vi "Build All VI HTML Documentation.vi"(6 "Requirement":string="Labstache", 7 "Destination":path=path "", 8 "Error In":errorcluster, 11 "Source In":path) -> (0 "Error Out":errorcluster, 3 "Source Out":path)   [LabVIEW 2018, in "Scripts.lvlib"]
uses:
  Scripts.lvlib
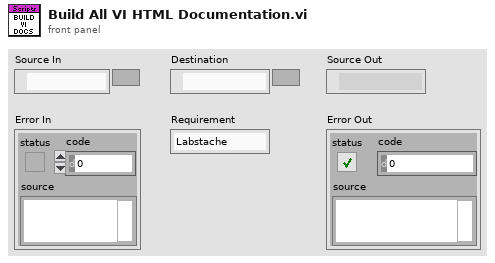
[diagram p1: front panel]
types:
  T1 = enum32{"invalid VI type", "Standard VI", "Control VI", "Global VI", "Polymorphic VI", "Configuration VI", "SubSystem", "Facade VI", "Method VI", "Statechart Diagram VI"}
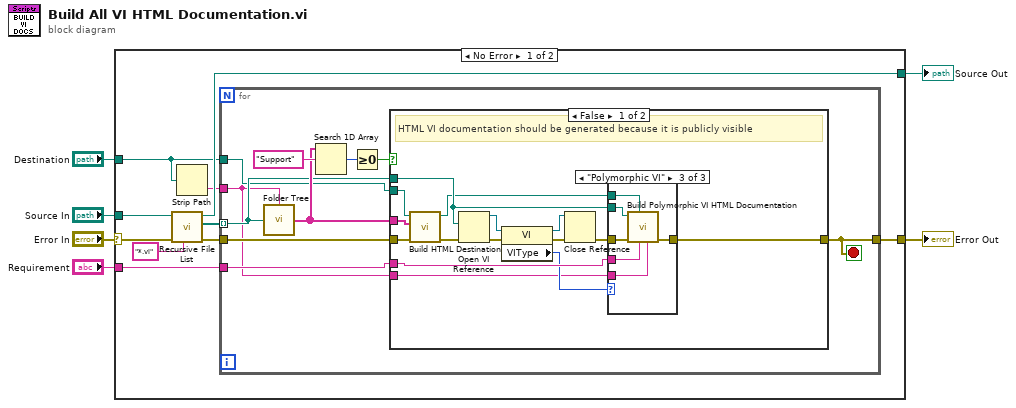
[diagram p0: block diagram]
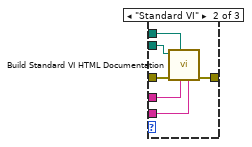
[diagram p3: hidden frame]
diagram:
  n1 = case shown="No Error" "Error In" {
    selector: "Error In" -> [w11 w57]
    tunnel: [w13 w57] -> w6
    tunnel: "Requirement" -> [w12 _]
    tunnel: "Destination" -> [w8 _]
    tunnel: "Source In" -> [w10 w56]
    tunnel: [w9 w56] -> w1
    frame No Error {
      n2 = call <vilib>:"Recursive File List.vi"("pattern"="*.vi", "error in (no error)"=w11, "Folder Path"=w10) -> ("error out"=w14:errorcluster, "All Files in Dir"=w15:path[], "dup Folder Path"=w9:path)  [unwired: 4 in, 2 out]
      n3 = Strip Path(path=w8) -> (name=w7:string)  [unwired: 1 out]
      n4 = for {
        tunnel: w15 -> [w20] mode=indexing
        tunnel: w14 -> [w22]
        tunnel: w7 -> [w18]
        tunnel: [w21] -> w13
        tunnel: w12 -> [w19]
        tunnel: w8 -> [w17]
        stop <- w21 stop-if-true
        n5 = call "Folder Tree.vi"("File"=w20, "Root Folder Name"=w18) -> ("Hierarchy Folders"=w23:string[])
        n6 = Search 1D Array(1D array=w23, element="Support") -> (index of element=w25:i32)  [unwired: 1 in]
        n7 = Greater Or Equal To 0?(x=w25) -> (x >= 0?=w24:bool)
        n8 = case shown="False" w24 {
          tunnel: w23 -> [w40 _]
          tunnel: w22 -> [w41 w55]
          tunnel: [w39 w55] -> w21
          tunnel: w20 -> [w33 _]
          tunnel: w19 -> [w38 _]
          tunnel: w18 -> [w30 _]
          tunnel: w17 -> [w29 _]
          frame False {
            # "HTML VI documentation should be generated because it is publicly visible"
            n9 = call "Build HTML Destination.vi"("Error In"=w41, "Hierarchy Folders"=w40, "Root Destination"=w29) -> ("Error Out"=w37:errorcluster, "HTML Destination"=w32:path)  [unwired: 7 in]
            n10 = Open VI Reference(vi path=w33, error in (no error)=w37) -> (vi reference=w36:refnum<vi>, error out=w35:errorcluster)  [unwired: 4 in]
            n11 = property class="VI"(reference=w36, error in=w35) -> (reference out=w27:refnum<vi>, error out=w28:errorcluster, "VIType"=w34:T1)
            n12 = Close Reference(reference=w27, error in (no error)=w28) -> (error out=w31:errorcluster)
            n13 = case shown="\"Polymorphic VI\"" w34 {
              tunnel: [w42 w48 w53] -> w39
              tunnel: w38 -> [_ w45 w50]
              tunnel: w33 -> [_ w47 w54]
              tunnel: w32 -> [_ w43 w51]
              tunnel: w31 -> [w42 w46 w52]
              tunnel: w30 -> [_ w44 w49]
              frame "invalid VI type", Default {
              }
              frame "Standard VI" {
                n14 = call "Build Standard VI HTML Documentation.vi"("Root Folder Name"=w44, "Requirement"=w45, "Destination"=w43, "Error In"=w46, "VI"=w47) -> ("Error Out"=w48:errorcluster)  [unwired: 6 in]
              }
              frame "Polymorphic VI" {
                n15 = call "Build Polymorphic VI HTML Documentation.vi"("Root Folder Name"=w49, "Requirement"=w50, "Destination"=w51, "Error In"=w52, "VI"=w54) -> ("Error Out"=w53:errorcluster)  [unwired: 6 in]
              }
            }
          }
          frame True {
            # "Is a private VI that does not need VI documentation generated"
          }
        }
      }
    }
    frame Error {
    }
  }
  "Error Out" <- w6
  "Source Out" <- w1
